vi "test_Import Bitfile Scalars_Label.vi"(8 "error in (no error)":errorcluster, 11 "TestCase in":refnum<class "FPGA Addon Scripting API Unit Tests.lvclass">) -> (0 "error out":errorcluster, 3 "TestCase out":refnum<class "FPGA Addon Scripting API Unit Tests.lvclass">)   [LabVIEW 2020, in "FPGA Addon Scripting API Unit Tests.lvclass"]
uses:
  FPGA Addon Scripting API Unit Tests.lvclass
  APIs/Scripting API/TypeDefs/Input Scalar Data.ctl
  APIs/Scripting API/TypeDefs/Output Scalar Data.ctl
  Addon/Addon Shared/Types/FPGA Addon Data Type.ctl
  APIs/Scripting API/Public/Bitfile Resources/Import Bitfile Scalars (Instances)/Import Scalars - by label.vi
  <vilib>/addons/_JKI Toolkits/VI Tester/TestCase.llb/TestCase.lvclass
  FPGA Addon Test Class/FPGA Addon Test Class.lvclass
  APIs/Scripting API/Scripting API.lvlib
  Addon/Addon Shared/FPGA Addon Shared.lvlib
  C:/Program Files (x86)/National Instruments/LabVIEW 2020/vi.lib/addons/_JKI Toolkits/VI Tester/TestCase.llb/TestCase.lvclass
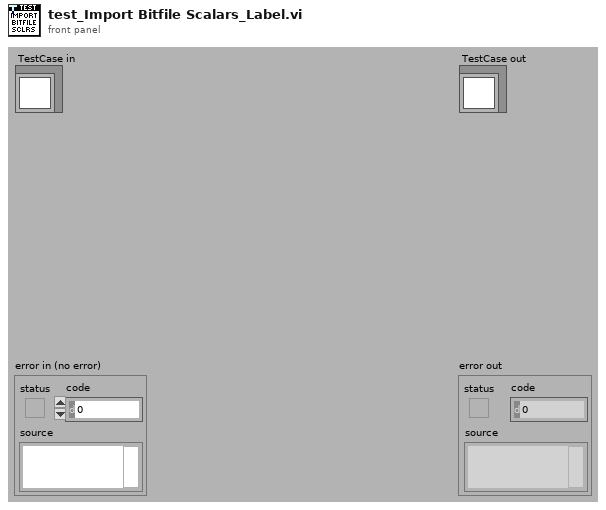
[diagram p1: front panel]
types:
  T1 = typedef "Scripting API.lvlib/Output Scalar Data.ctl" = cluster{"Bitfile Name":string, "SysDef Channel Name":string, "Imported":bool, "Data Type":T2}
  T2 = typedef "FPGA Addon Shared.lvlib/FPGA Addon Data Type.ctl" = enum8{"<Null>", "I8", "I16", "I32", "I64", "U8", "U16", "U32", "U64", "SGL", "Boolean", "Analog PWM In Settings", "Analog PWM In", "Digital PWM In Settings", "Digital PWM In", "Digital PWM Out", "Sine Out", "FXP", "FXP+/-24.5", "FXP+/-16.5", "FXP+/-32.8", "FXP+/-64.32", "FXP+/-16.7", "FXP+/-20.5", "FXP+/-27.5", "FXP+/-32.16", "FXP+16.3", "FXP+18.3", "Digital Static In", "Digital Static Out", "Digital Static In Settings", "Digital WSS Out", "Quad Encoder Settings", "Quad Encoder In", "Group"}
  T3 = typedef "Scripting API.lvlib/Input Scalar Data.ctl" = cluster{"Bitfile Name":string, "SysDef Name":string}
  T4 = typedef "Custom Device API.lvlib/Custom Device Item Ref.ctl" = u64
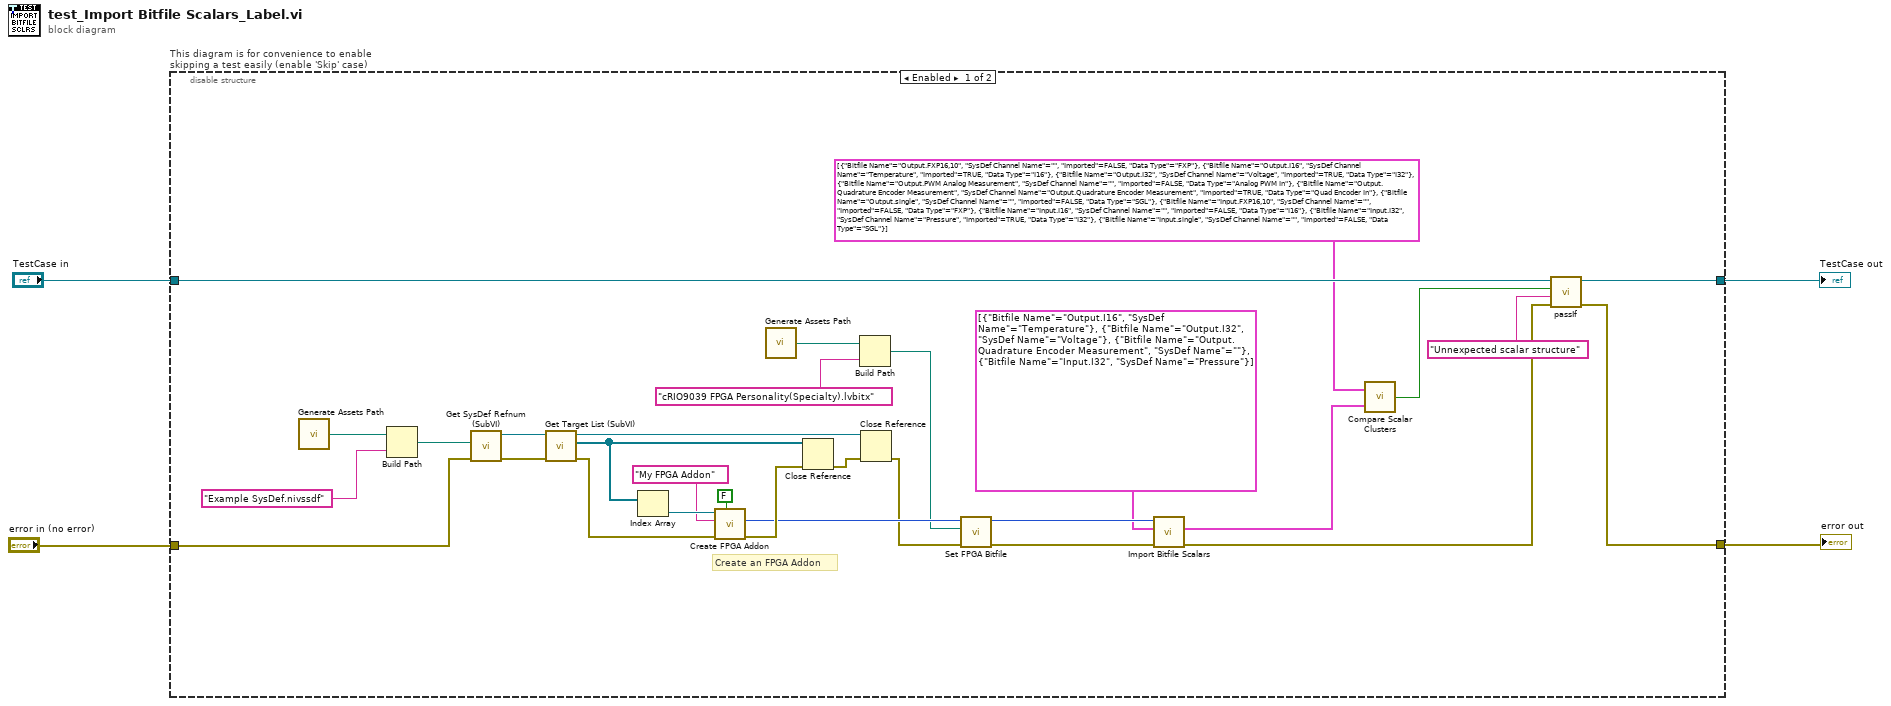
[diagram p0: block diagram]
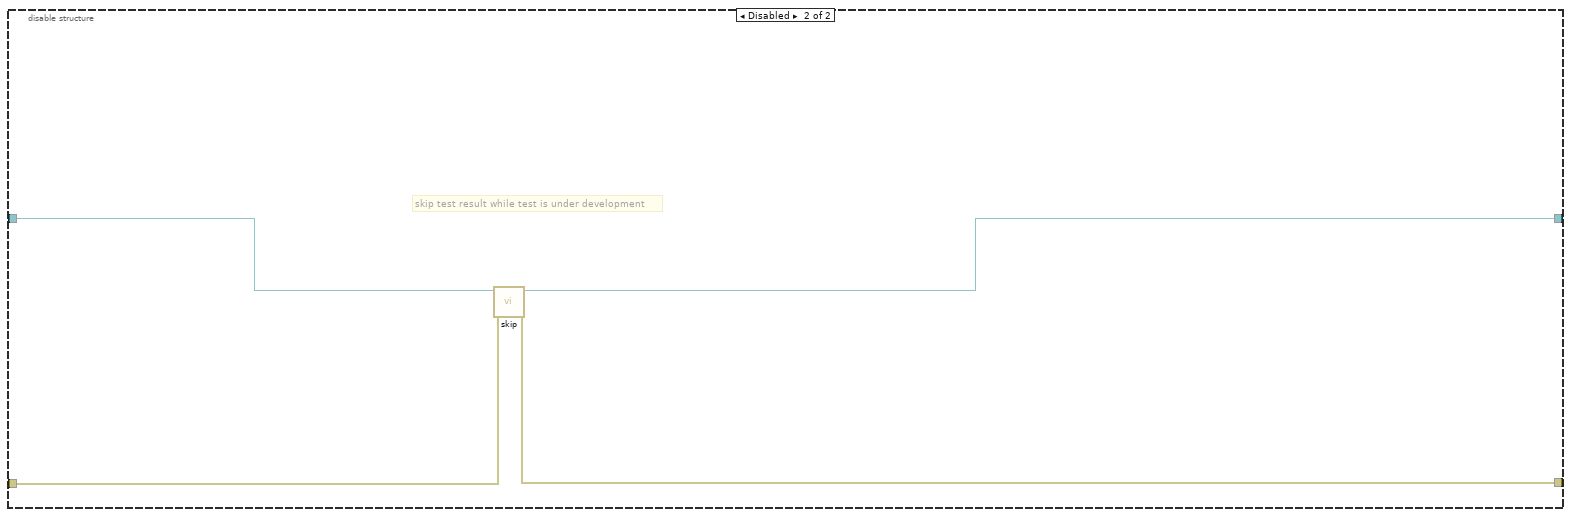
[diagram p2: hidden frame]
diagram:
  n1 = disable-structure "This diagram is for convenience to enable skipping a test easily (enable 'Skip' case)" shown="Enabled" {
    disable-tunnel: "TestCase in" -> [w10 w38]
    disable-tunnel: [w9 w36] -> w1
    disable-tunnel: [w8 w37] -> w3
    disable-tunnel: "error in (no error)" -> [w28 w35]
    frame Enabled {
      # "Create an FPGA Addon"
      n2 = call "Generate Assets Path.vi"() -> ("Assets path"=w34:path)
      n3 = Build Path(base path=w34, name or relative path="Example SysDef.nivssdf") -> (appended path=w32:path)
      n4 = call "Get SysDef Refnum (SubVI).vi"("error in (no error)"=w28, "System Definition path"=w32) -> ("error out"=w27:errorcluster, "SysDef Refnum out"=w31:refnum<k24>)  [unwired: 8 in]
      n5 = call "Get Target List (SubVI).vi"("error in (no error)"=w27, "SysDef Refnum in"=w31) -> ("error out"=w26:errorcluster, "Target List Refnums"=w25:refnum<k24>[], "SysDef Refnum out"=w24:refnum<k24>)  [unwired: 7 in]
      n6 = Index Array(array=w25) -> (element=w30:refnum<k24>)  [unwired: 1 in]
      n7 = call "Create FPGA Addon.vi"("group scalars"=FALSE, "error in"=w26, "FPGA addon name"="My FPGA Addon", "target in"=w30) -> ("error out"=w22:errorcluster, "FPGA addon refnum"=w20:T4)  [unwired: 5 in, 1 out]
      n8 = call "Generate Assets Path.vi"() -> ("Assets path"=w18:path)
      n9 = Close Reference(reference=w25, error in (no error)=w22) -> (error out=w23:errorcluster)
      n10 = Build Path(base path=w18, name or relative path="cRIO9039 FPGA Personality(Specialty).lvbitx") -> (appended path=w16:path)
      n11 = Close Reference(reference=w24, error in (no error)=w23) -> (error out=w19:errorcluster)
      n12 = call "Set FPGA Bitfile.vi"("error in"=w19, "FPGA bitfile path"=w16, "FPGA addon refnum in"=w20) -> ("error out"=w15:errorcluster, "FPGA addon refnum out"=w14:T4)  [unwired: 7 in]
      n13 = call-poly "Import Bitfile Scalars.vi"("error in"=w15, "bitfile scalars in"=T3[] [{"Bitfile Name"="Output.I16", "SysDef Name"="Temperature"}, {"Bitfile Name"="Output.I32", "SysDef Name"="Voltage"}, {"Bitfile Name"="Output.Quadrature Encoder Measurement", "SysDef Name"=""}, {"Bitfile Name"="Input.I32", "SysDef Name"="Pressure"}], "FPGA addon refnum in"=w14) -> ("error out"=w11:errorcluster, "imported bitfile scalars out"=w12:T1[])  [unwired: 6 in, 1 out]
      n14 = call "Compare Scalar Clusters.vi"("Target bitfile scalars in"=w12, "Reference bitfile scalars in"=T1[] [{"Bitfile Name"="Output.FXP16,10", "SysDef Channel Name"="", "Imported"=FALSE, "Data Type"=enum."FXP"}, {"Bitfile Name"="Output.I16", "SysDef Channel Name"="Temperature", "Imported"=TRUE, "Data Type"=enum."I16"}, {"Bitfile Name"="Output.I32", "SysDef Channel Name"="Voltage", "Imported"=TRUE, "Data Type"=enum."I32"}, {"Bitfile Name"="Output.PWM Analog Measurement", "SysDef Channel Name"="", "Imported"=FALSE, "Data Type"=enum."Analog PWM In"}, {"Bitfile Name"="Output.Quadrature Encoder Measurement", "SysDef Channel Name"="Output.Quadrature Encoder Measurement", "Imported"=TRUE, "Data Type"=enum."Quad Encoder In"}, {"Bitfile Name"="Output.single", "SysDef Channel Name"="", "Imported"=FALSE, "Data Type"=enum."SGL"}, {"Bitfile Name"="Input.FXP16,10", "SysDef Channel Name"="", "Imported"=FALSE, "Data Type"=enum."FXP"}, {"Bitfile Name"="Input.I16", "SysDef Channel Name"="", "Imported"=FALSE, "Data Type"=enum."I16"}, {"Bitfile Name"="Input.I32", "SysDef Channel Name"="Pressure", "Imported"=TRUE, "Data Type"=enum."I32"}, {"Bitfile Name"="Input.single", "SysDef Channel Name"="", "Imported"=FALSE, "Data Type"=enum."SGL"}] ("imported bitfile scalars out")) -> ("Equal ?"=w7:bool)
      n15 = call-dynamic "passIf.vi"("error in (no error)"=w11, "message (\"\")"="Unnexpected scalar structure" ("message (\"\")"), "pass"=w7, "TestCase in"=w10) -> ("error out"=w8:errorcluster, "TestCase out"=w9:refnum<class "FPGA Addon Scripting API Unit Tests.lvclass">)  [unwired: 6 in]
    }
    frame Disabled {
      # "skip test result while test is under development"
      n16 = call <vilib>:"skip.vi"("error in (no error)"=w35, "TestCase in"=w38) -> ("error out"=w37:errorcluster, "TestCase out"=w36:refnum<class "FPGA Addon Scripting API Unit Tests.lvclass">)  [unwired: 8 in]
    }
  }
  "error out" <- w3
  "TestCase out" <- w1
